vi "INI read triggering.vi"(8 "error in (no error)":T4, 11 "Port":string(combo)="tx") -> (0 "error out":T4, 2 "Trig opt":T1 {"delay" format="%.3p"}, 3 "Port out":string(combo)="tx")   [LabVIEW 2019, in "Shared.lvlib"]
uses:
  Shared.lvlib
  Low-level/TypeDefs/TX trigger config.ctl
  FPGA/SubVIs/Utility/FPGA driver trigger source.ctl
  FPGA/SubVIs/Utility/FPGA driver trigger destination.ctl
  System GV.vi
  <vilib>/Utility/config.llb/NI_LVConfig.lvlib
  FPGA/SubVIs/Utility/FPGA Utility.lvlib
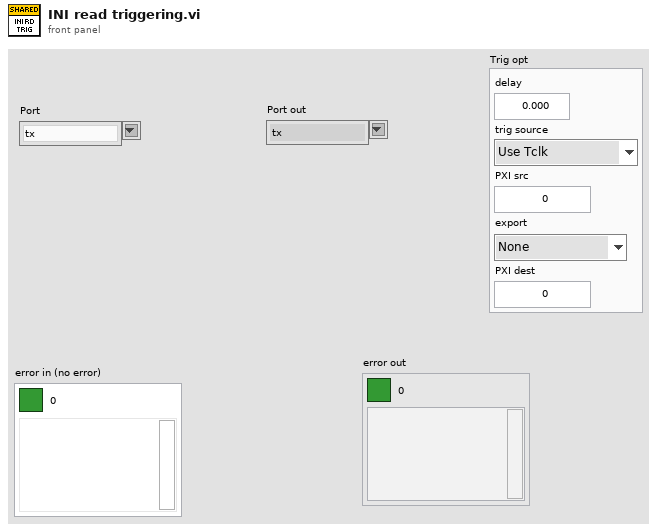
[diagram p1: front panel]
types:
  T1 = typedef "TX trigger config.ctl" = cluster{"delay":dbl, "trig source":T2, "PXI src":i32, "export":T3, "PXI dest":i32}
  T2 = typedef "FPGA Utility.lvlib/FPGA driver trigger source.ctl" = enum16{"Use Tclk", "PXI_Trig", "Aurora RX trig"}
  T3 = typedef "FPGA Utility.lvlib/FPGA driver trigger destination.ctl" = enum16{"None", "Source trig", "Synced trig", "Delayed sync"}
  T4 = cluster{"Boolean Round":bool, "code":i32, "source":string}
  T5 = cluster{"TX_delay":dbl, "TX_trig_src":T2, "TX_PXI_src":i32, "TX_export":T3, "TX_PXI_dest":i32, "RX_delay":dbl, "RX_trig_src":T2, "RX_PXI_src":i32, "RX_export":T3, "RX_PXI_dest":i32}
  T6 = typedef "NI_LVConfig.lvlib/Config Data RefNum.ctl" = refnum<k1>
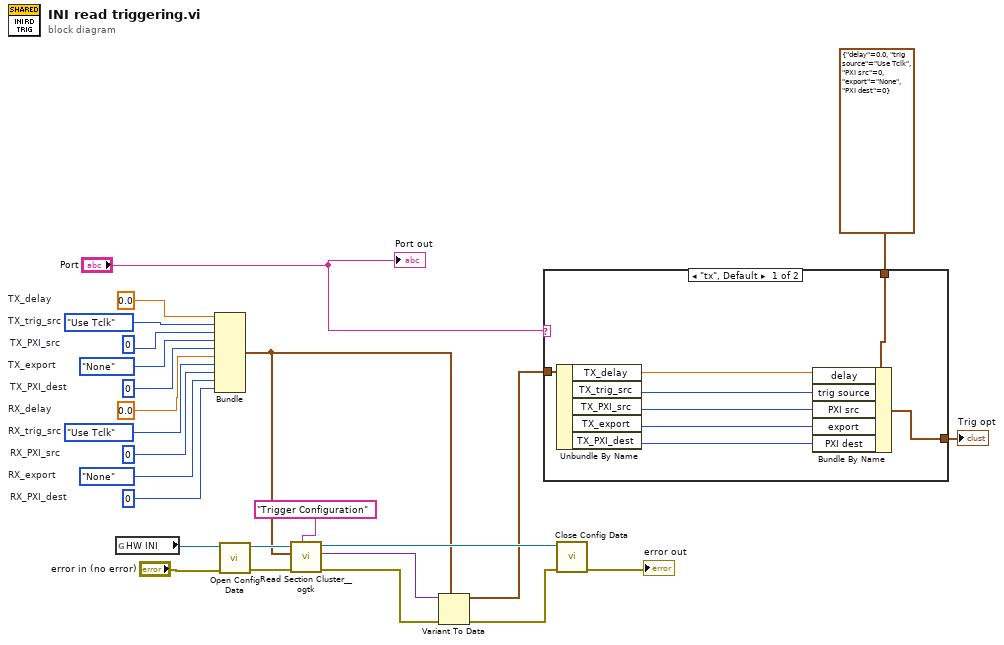
[diagram p0: block diagram]
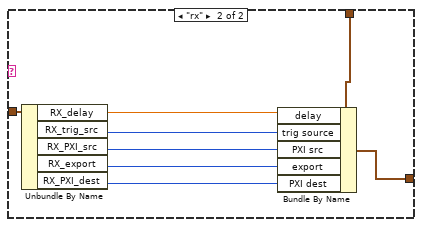
[diagram p2: hidden frame]
diagram:
  w2 = 0  # RX_PXI_dest
  w4 = 0  # RX_PXI_src
  w3 = FPGA_driver_trigger_destination."None"  # RX_export
  w5 = FPGA_driver_trigger_source."Use Tclk"  # RX_trig_src
  w6 = 0.0  # RX_delay
  w7 = 0  # TX_PXI_dest
  w9 = 0  # TX_PXI_src
  w8 = FPGA_driver_trigger_destination."None"  # TX_export
  w10 = FPGA_driver_trigger_source."Use Tclk"  # TX_trig_src
  w13 = 0.0  # TX_delay
  n1 = global read "System GV.vi" "HW INI"() -> (w22:path)
  n2 = Bundle("TX_delay"=w13, "TX_trig_src"=w10, "TX_PXI_src"=w9, "TX_export"=w8, "TX_PXI_dest"=w7, "RX_delay"=w6, "RX_trig_src"=w5, "RX_PXI_src"=w4, "RX_export"=w3, "RX_PXI_dest"=w2) -> (w17:T5)  [unwired: 1 in]
  n3 = call <vilib>:"Open Config Data.vi"("error in (no error)"="error in (no error)", "configuration file path"=w22) -> ("error out"=w23:errorcluster, "refnum"=w25:T6)  [unwired: 7 in, 1 out]
  n4 = call <userlib>:"Read Section Cluster__ogtk.vi"("section (optional)"="Trigger Configuration", "error in (no error)"=w23, "Section Formatted Cluster Type"=w17, "refnum"=w25) -> ("error out"=w19:errorcluster, "Section Formatted Cluster"=w20:variant, "dup refnum"=w24:T6)  [unwired: 3 in, 2 out]
  n5 = Variant To Data(error in=w19, type=w17, Variant=w20) -> (data=w16:T5, error out=w18:errorcluster)
  n6 = case shown="\"tx\", Default" "Port" {
    tunnel: w16 -> [w32 w40]
    tunnel: [w31 w39] -> w1
    tunnel: T1 {"delay"=0.0, "trig source"=enum."Use Tclk", "PXI src"=0, "export"=enum."None", "PXI dest"=0} ("TX trigger options") -> [w33 w41]
    frame "tx", Default {
      n7 = Unbundle By Name(w32) -> ("TX_delay"=w26:dbl, "TX_trig_src"=w30:T2, "TX_PXI_src"=w29:i32, "TX_export"=w28:T3, "TX_PXI_dest"=w27:i32)
      n8 = Bundle By Name(cluster=w33, "delay"=w26, "trig source"=w30, "PXI src"=w29, "export"=w28, "PXI dest"=w27) -> (w31:T1)
    }
    frame "rx" {
      n9 = Unbundle By Name(w40) -> ("RX_delay"=w34:dbl, "RX_trig_src"=w38:T2, "RX_PXI_src"=w37:i32, "RX_export"=w36:T3, "RX_PXI_dest"=w35:i32)
      n10 = Bundle By Name(cluster=w41, "delay"=w34, "trig source"=w38, "PXI src"=w37, "export"=w36, "PXI dest"=w35) -> (w39:T1)
    }
  }
  "Trig opt" <- w1
  n11 = call <vilib>:"Close Config Data.vi"("error in (no error)"=w18, "refnum"=w24) -> ("error out"=→"error out":errorcluster)  [unwired: 8 in, 1 out]
  "Port out" <- "Port"
